vi "controlGroundAxis.vi"(7 "set":bool, 8 "error in":errorcluster, 9 "groundAxis in":bool, 10 "axis":i32, 11 "connection ID":i32) -> (0 "error out":errorcluster, 2 "axis_out":i32, 3 "connection ID":i32)   [LabVIEW 2016]
panel:
  out "groundAxis out":bool
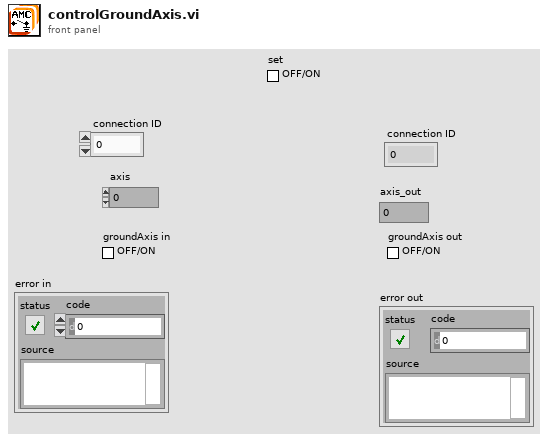
[diagram p1: front panel]
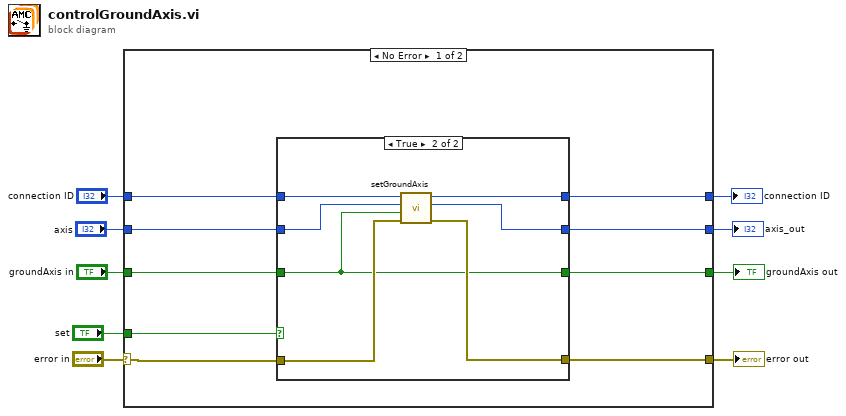
[diagram p0: block diagram]
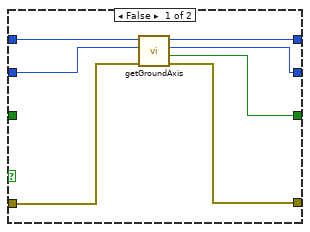
[diagram p2: hidden frame]
diagram:
  n1 = case shown="No Error" "error in" {
    selector: "error in" -> [w15 w36]
    tunnel: [w14 w36] -> w9
    tunnel: [w17 w35] -> w8
    tunnel: "connection ID" -> [w18 w35]
    tunnel: "axis" -> [w13 w33]
    tunnel: "set" -> [w16 _]
    tunnel: "groundAxis in" -> [w12 w34]
    tunnel: [w11 w34] -> w2
    tunnel: [w10 w33] -> w1
    frame No Error {
      n2 = case shown="True" w16 {
        tunnel: w18 -> [w25 w32]
        tunnel: [w24 w31] -> w17
        tunnel: w15 -> [w23 w30]
        tunnel: [w22 w29] -> w14
        tunnel: w13 -> [w20 w28]
        tunnel: w12 -> [_ w27]
        tunnel: [w21 w27] -> w11
        tunnel: [w19 w26] -> w10
        frame False {
          n3 = call "getGroundAxis.vi"("error in"=w23, "axis"=w20, "connection ID"=w25) -> ("error out"=w22:errorcluster, "grounded"=w21:bool, "axis_out"=w19:i32, "connection ID"=w24:i32)  [unwired: 5 in]
        }
        frame True {
          n4 = call "setGroundAxis.vi"("error in"=w30, "enabled"=w27, "axis"=w28, "connection ID"=w32) -> ("error out"=w29:errorcluster, "axis_out"=w26:i32, "connection ID"=w31:i32)  [unwired: 5 in]
        }
      }
    }
    frame Error {
    }
  }
  "error out" <- w9
  "connection ID" <- w8
  "axis_out" <- w1
  "groundAxis out" <- w2
